vi "unused_Write loopCounter.vi"(8 "error in (no error)":errorcluster, 10 "loopCounter":i32, 11 "ExampleTask_StopNotifier in":refnum<class "ExampleTask_BoolUserEventStopNotifier.lvclass">) -> (0 "error out":errorcluster, 3 "ExampleTask_StopNotifier out":refnum<class "ExampleTask_BoolUserEventStopNotifier.lvclass">)   [LabVIEW 2023]
uses:
  ExampleTask_BoolUserEventStopNotifier.lvclass
  ExampleTask_BoolUserEventStopNotifier.lvclass/ExampleTask_BoolUserEventStopNotifier.ctl
  C:/projects/TLC_Daemon/source/Examples/ExampleTask_BoolUserEventStopNotifier/ExampleTask_BoolUserEventStopNotifier.lvclass
  C:/projects/TLC_Daemon/source/ITask/ITask.lvclass
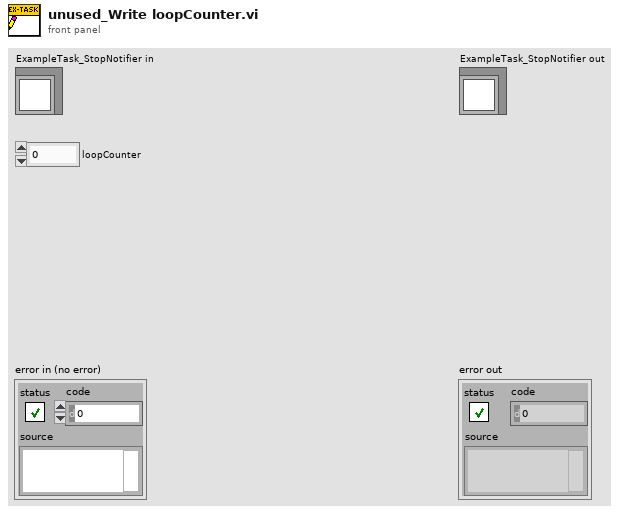
[diagram p1: front panel]
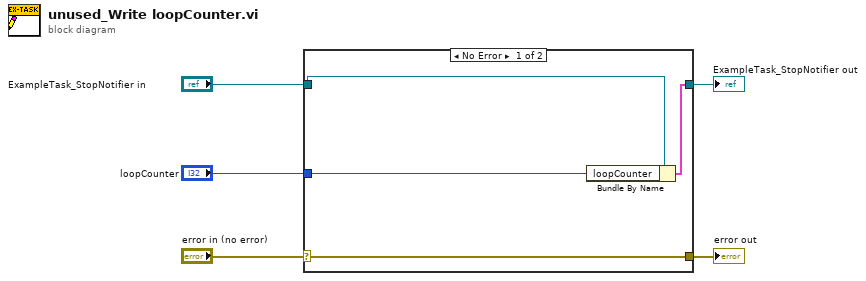
[diagram p0: block diagram]
diagram:
  n1 = case shown="No Error" "error in (no error)" {
    selector: "error in (no error)" -> [w9 w10]
    tunnel: [w9 w10] -> w4
    tunnel: [w7 w11] -> w2
    tunnel: "ExampleTask_StopNotifier in" -> [w8 w11]
    tunnel: "loopCounter" -> [w6 _]
    frame No Error {
      n2 = Bundle By Name(cluster=w8, "loopCounter"=w6) -> (w7:cluster{})
    }
    frame Error {
    }
  }
  "error out" <- w4
  "ExampleTask_StopNotifier out" <- w2
